vi "Untitled 1.vi"() -> ()   [LabVIEW 2019]
panel:
  out "third row fifth col":dbl
  in  "Row":i32
  in  "Column":i32
  out "Second Col":dbl[](array[numeric])
  out "Third Row":dbl[](array[numeric])
  out "Array":dbl[][](array[numeric])
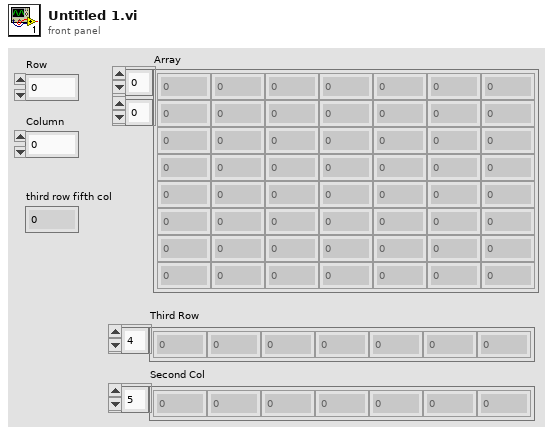
[diagram p1: front panel]
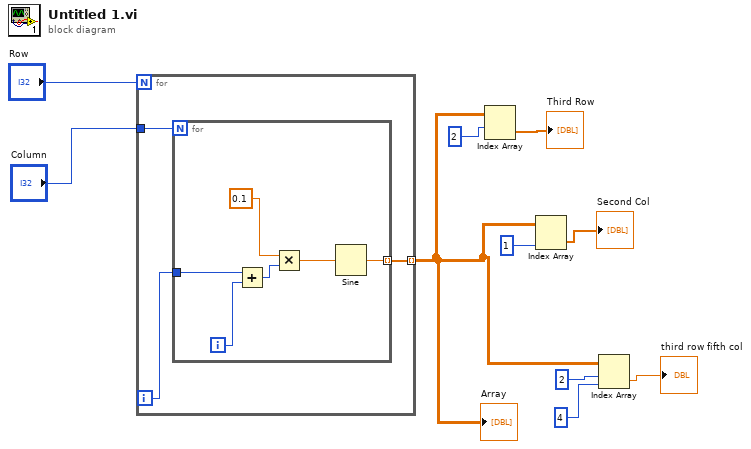
[diagram p0: block diagram]
diagram:
  n1 = for {
    N: "Row" -> [_]
    tunnel: "Column" -> [w12]
    tunnel: [w11] -> w4 mode=indexing
    i -> [w13]
    n2 = for {
      N: w12 -> [_]
      tunnel: w13 -> [w19]
      tunnel: [w15] -> w11 mode=indexing
      i -> [w18]
      n3 = Add(x=w19, y=w18) -> (x+y=w14:i32)
      n4 = Multiply(x=0.1, y=w14) -> (x*y=w16:dbl)
      n5 = Sine(x=w16) -> (sin(x)=w15:dbl)
    }
  }
  "Array" <- w4
  n6 = Index Array(array=w4, index (row)=2) -> (element=→"Third Row":dbl[])  [unwired: 1 in]
  n7 = Index Array(array=w4, index (col)=1) -> (element=→"Second Col":dbl[])  [unwired: 1 in]
  n8 = Index Array(array=w4, index (row)=2 ("disabled index (row)"), index (col)=4) -> (element=→"third row fifth col":dbl)
